vi "Bodies_GetUnitVecInXYZ0.vi"(8 "error in (no error)":errorcluster, 9 "Dir of Vector":T1, 10 "Body ID":i32, 11 "Bodies.lvclass":refnum<class "Bodies.lvclass">) -> (0 "error out":errorcluster, 2 "UnitVec in GCS":dbl[](array[numeric]) format="%#.6f", 3 "Bodies.lvclass 2":refnum<class "Bodies.lvclass">)   [LabVIEW 2015, in "Bodies.lvclass"]
doc: "Find the unit vector of ith body in GLOBAL frame. X,Y,Y will give unit vector of the that direction, and O will give the the joint center coordinate."
uses:
  Bodies.lvclass
  xyzO.ctl
  Bodies.lvclass/Bodies.ctl
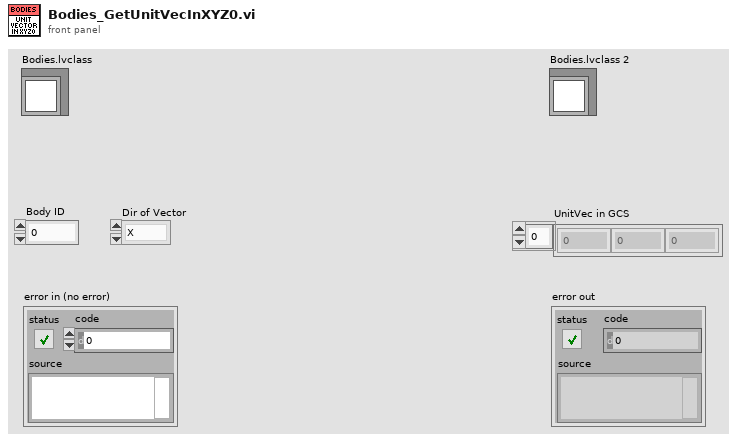
[diagram p1: front panel]
types:
  T1 = typedef "Bodies.lvclass/xyzO.ctl" = enum16{"X", "Y", "Z", "O"}
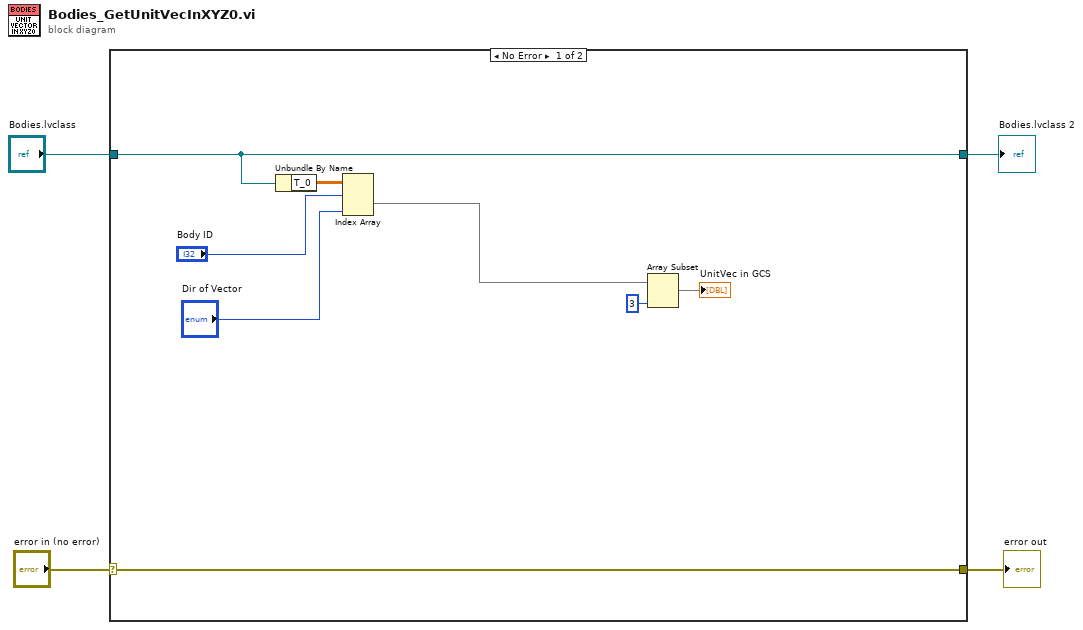
[diagram p0: block diagram]
diagram:
  n1 = case shown="No Error" "error in (no error)" {
    selector: "error in (no error)" -> [w7 w14]
    tunnel: "Bodies.lvclass" -> [w5 w13]
    tunnel: [w7 w14] -> w3
    tunnel: [w5 w13] -> w1
    frame No Error {
      n2 = Unbundle By Name(w5) -> ("T_0"=w6:dbl[][][])
      n3 = Index Array(array=w6, index (dim 0)="Body ID", index (dim 2)="Dir of Vector") -> (element=w8:dbl[])  [unwired: 1 in]
      n4 = Array Subset(array=w8, length=3) -> (→"UnitVec in GCS":dbl[])  [unwired: 1 in]
    }
    frame Error {
    }
  }
  "error out" <- w3
  "Bodies.lvclass 2" <- w1
